vi "Support_Top_Level.vi"(8 "error in (no error)":errorcluster, 11 "AB_Dest_App in":refnum<class "AB_Dest_LegacyApp.lvclass">) -> (0 "error out":errorcluster, 1 "displayTopLevel":bool, 2 "supportTopLevel":bool, 3 "AB_Dest_App out":refnum<class "AB_Dest_LegacyApp.lvclass">)   [LabVIEW 2020, in "AB_Dest_LegacyApp.lvclass"]
uses:
  <vilib>/AppBuilder/AB_Classes/Destination/Dest_LegacyApplication/AB_Dest_LegacyApp.lvclass
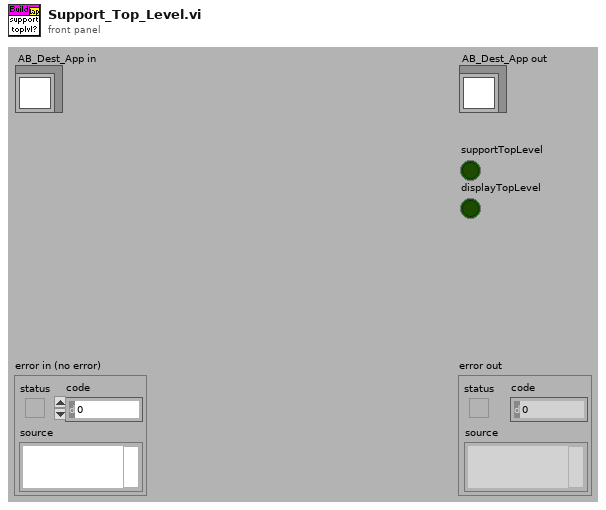
[diagram p1: front panel]
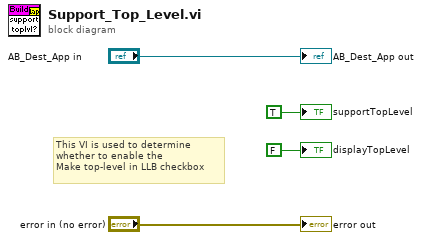
[diagram p0: block diagram]
diagram:
  # "This VI is used to determine\nwhether to enable the \nMake top-level in LLB checkbox"
  "error out" <- "error in (no error)"
  "supportTopLevel" <- TRUE ("supportTopLevel")
  "AB_Dest_App out" <- "AB_Dest_App in"
  "displayTopLevel" <- FALSE ("supportTopLevel")
